vi "MS Auto Operation.vi"() -> ()   [LabVIEW 2016]
uses:
  <vilib>/rvi/interface/nirviReadWriteControl/nirviReadWriteControl.xnode
  <vilib>/rvi/interface/nirviOpenFPGA/nirviOpenFPGA.xnode
  <vilib>/rvi/interface/nirviCloseFPGA/nirviCloseFPGA.xnode
  <vilib>/rvi/interface/nirviMethod/nirviMethod.xnode
  Subsystems/Global Variables.vi
  <vilib>/Analysis/Matrix/Datatypes/RealMatrix.ctl
  <vilib>/Analysis/Matrix/NI_Matrix.lvlib
  NiFpgaLv.dll
  <vilib>/Utility/error.llb/Error Cluster From Error Code.vi
  <vilib>/rvi/errors/niLvFpgaAdjustHostInterfaceError.vi
  IRISS_FPGA_IO_RIO.vi
  FPGA Bitfiles/IRISSTrack_FPGATarget2_IRISSFPGAIORIO_4NTO9ubhv-c.lvbitx
  <vilib>/FPGAPlugInAG/myRIO-1900/niLvFpga_Open_myRIO-1900.vi
  <vilib>/FPGAPlugInAG/myRIO-1900/niLvFpga_Reset_myRIO-1900.vi
  <vilib>/FPGAPlugInAG/myRIO-1900/niLvFpga_Close_myRIO-1900.vi
panel:
  out "Stage PID Cluster":T1={"Stage Z PID"={"Kp"=0.0005, "Kd"=0.001, "Ki"=0.0}, "Stage Y PID"={"Kp"=0.0003, "Kd"=0.01, "Ki"=0.0}, "Stage X PID"={"Kp"=0.0003, "Kd"=0.01, "Ki"=0.0}}
  out "L1 to L4 PID Cluster":T2={"L1 PID Gains"={"Kp"=0.005, "Kd"=0.5, "Ki"=0.0005}, "L2 PID Gains"={"Kp"=0.01, "Kd"=1.0, "Ki"=0.0005}, "L3 PID Gains"={"Kp"=0.05, "Kd"=1.0, "Ki"=0.0005}, "L4 PID Gains"={"Kp"=0.1, "Kd"=1.0, "Ki"=0.0005}}
  in  "IRISS GUI":T3(tab)
  in  "Reroute Hold [sec]":dbl=10.0 caption="Hold [sec]"
  out "X Stage out [mm] 2":dbl caption="Stage X [mm]" format="%#.4f"
  out "Z Stage out [mm] 2":dbl caption="Stage Z [mm]" format="%#.4f"
  out "Y Stage out [mm] 2":dbl caption="Stage Y [mm]" format="%#.4f"
  in  "Refractice Index":dbl=1.35
  out "Asgn Pt Out of Bound":bool caption="Assign Pt OOB"
  out "Finished Late Counts":u16
  out "Emergency alarm":bool
  out "Remote sender engaged":bool
  in  "L2 PID Gains":cluster{"Kp":dbl, "Kd":dbl, "Ki":dbl}={"Kp"=0.01, "Kd"=1.0, "Ki"=0.005}
  in  "L3 PID Gains":cluster{"Kp":dbl, "Kd":dbl, "Ki":dbl}={"Kp"=0.05, "Kd"=1.0, "Ki"=0.0005}
  in  "L4 PID Gains":cluster{"Kp":dbl, "Kd":dbl, "Ki":dbl}={"Kp"=0.1, "Kd"=0.1, "Ki"=0.0005}
  in  "L1 PID Gains":cluster{"Kp":dbl, "Kd":dbl, "Ki":dbl}={"Kp"=0.01, "Kd"=0.5, "Ki"=0.001}
  out "Current System State":T4(ring)
  out "State changing":bool
  out "Current Run No.":u8
  out "Tip out Posit":dbl[](array[numeric]) caption="Position [mm]" format="%#.3f"
  out "Tip cmd Posit":dbl[](array[numeric]) caption="Command [mm]" format="%#.3f"
  out "L4 out Posit":dbl caption="y [deg]" format="%#.2g"
  out "L4 cmd Posit":dbl caption="r [deg]" format="%#.2g"
  out "L3 out Posit":dbl caption="y [mm]" format="%#.2g"
  out "L3 cmd Posit":dbl caption="r [mm]" format="%#.2g"
  out "L2 out Posit":dbl caption="y [deg]" format="%#.2g"
  out "L2 cmd Posit":dbl caption="r [deg]" format="%#.2g"
  out "L1 out Posit":dbl caption="y [deg]" format="%#.2g"
  out "L1 cmd Posit":dbl caption="r [deg]" format="%#.2g"
  out "State Flag Array":bool[](array[boolean])
  out "Timer":i32 format="%<%M:%S>t"
  out "Elaspsed Time":sgl
  in  "File Path":path=path "C:/KevData1.txt"
  in  "Seconds of Data":sgl=5.0
  out "Period [ms]":i64=10
  in  "Remote Control Source":u16(ring) caption="Remote Source" items=["Surgical Console", "Joystick"]
  in  "Reset Joystick":bool caption="Encoder Reset"
  in  "Robot Command":dbl[](array[numeric])=[0.0, 0.0, 0.0, 0.0]
  out "Z Stage out [mm]":dbl caption="Output Z [mm]" format="%#.4f"
  out "Z Stage cmd [mm]":dbl=6.0 caption="Reference Z [mm]" min=0.0 max=12.0 step=0.5
  out "Y Stage out [mm]":dbl caption="Output Y [mm]" format="%#.4f"
  out "Y Stage cmd [mm]":dbl=6.0 caption="Reference Y  [mm]" min=0.0 max=12.0 step=0.5
  out "X Stage out [mm]":dbl caption="Output X [mm]" format="%#.4f"
  out "X Stage cmd [mm]":dbl=6.0 caption="Reference X [mm]" min=0.0 max=12.0 step=0.5
  in  "Stage Z PID Gains":cluster{"Kp":dbl, "Kd":dbl, "Ki":dbl}={"Kp"=0.0005, "Kd"=0.001, "Ki"=0.0}
  in  "Stage Y PID Gains":cluster{"Kp":dbl, "Kd":dbl, "Ki":dbl}={"Kp"=0.0001, "Kd"=0.005, "Ki"=0.0}
  in  "Stage X PID Gains":cluster{"Kp":dbl, "Kd":dbl, "Ki":dbl}={"Kp"=0.0003, "Kd"=0.01, "Ki"=0.0}
  in  "Reroute Transit Vacf":dbl=100.0
  in  "Z Rot Axis":dbl=1.0
  in  "Z Dist Thld":dbl[](array[numeric])=[0.5, 2.0] caption="Z Distance Threshould"
  in  "Vac Extremum":dbl[](array[numeric])=[80.0, 100.0] caption="Vacuum Extremum"
  in  "Min PC Gap":dbl=0.1 caption="Min PC Gap [mm]" min=0.0 max=10.0 step=0.1 format="%#.3g"
  in  "Min AC Gap":dbl=0.1 caption="Min AC Gap [mm]" min=0.0 max=10.0 step=0.1 format="%#.3g"
  in  "Joint Limits":dbl[][](array[numeric])=[[-8.0, 35.0], [-35.0, 35.0], [-5.0, 10.0], [-180.0, 180.0]] format="%#.3g"
  in  "Offset Home 2 RCM":dbl[](array[numeric])=[-7.7, 37.0, 55.0, 0.0] format="%#.3g"
  out "Error(s) Out on Program End":errorcluster
  out "L4 Waveform Graph":dbl[](graph)
  out "L3 Waveform Graph":dbl[](graph)
  out "L2 Waveform Graph":dbl[](graph)
  out "L1 Waveform Graph":dbl[](graph)
  in  "Aiming Pt":dbl[](array[numeric])=[10.0, 0.0, -1.0, 0.0] format="%#.3g"
  in  "Engage Pt":dbl[](array[numeric])=[15.0, 0.0, 3.0, 0.0] format="%#.3g"
  in  "Inc Ctrl":dbl[](array[numeric])=[0.1, 0.05, 0.05] caption="Increment Control"
  in  "L3 Go Home":bool caption="To M/S"
  in  "Program Stop":bool
  # "M/S\n\nAuto"
  # "Robot Status"
  # "Tool Tip Location"
  # "Tracking Planning"
  # "L1"
  # "X\nY\nZ"
  # "X\nY\nZ"
  # "L2"
  # "System Progress"
  # "Assign Point Rerouting"
  # "X\nY\nZ"
  # "L3"
  # "Homing finished"
  # "M/S initialization finished"
  # "Tool Cruising Boundaries"
  # "Trajecoty loading finished"
  # "XY-plane"
  # "Z-axis"
  # "Aiming finished"
  # "L4"
  # "Tool engaged"
  # "Tracking initialization finished"
  # "In Tracking"
  # "Rerouting finished"
  # "In regulation"
  # "Vacuum"
  # "X\nY"
  # "X\nY"
  # "L1"
  # "L2"
  # "L3"
  # "L4"
  # "Data Saving"
  # "IOP Feedback Control"
  # "XYZ Stage Control"
  # "OCT Z-Axis"
  # "Foot Pedal Buttons"
  # "Irrigation and Aspiration"
  # "Button 1"
  # "Button 2"
  # "Button 3"
  # "Rotation & Vacuum Force Scheduling"
  # "Joint Motion & Control"
  # "Calibration"
  # "Space Deform Parameters"
  # "L1"
  # "[deg]"
  # "S"
  # "L2"
  # "[deg]"
  # "R"
  # "[deg]"
  # "L3"
  # "[mm]"
  # "T"
  # "[mm]"
  # "L4"
  # "[deg]"
  # "First Track Point"
  # "AC & PC Gap"
  # "L1"
  # "[deg]"
  # "L2"
  # "[deg]"
  # "L3"
  # "[mm]"
  # "L4"
  # "[deg]"
  # "Error Message"
  # "Tracking Joint Limits"
  # "Incision"
  # "Min."
  # "Max."
  # "L1"
  # "L1"
  # "[deg]"
  # "L2"
  # "L2"
  # "[deg]"
  # "L3"
  # "L3"
  # "[mm]"
  # "L4"
  # "L4"
  # "[deg]"
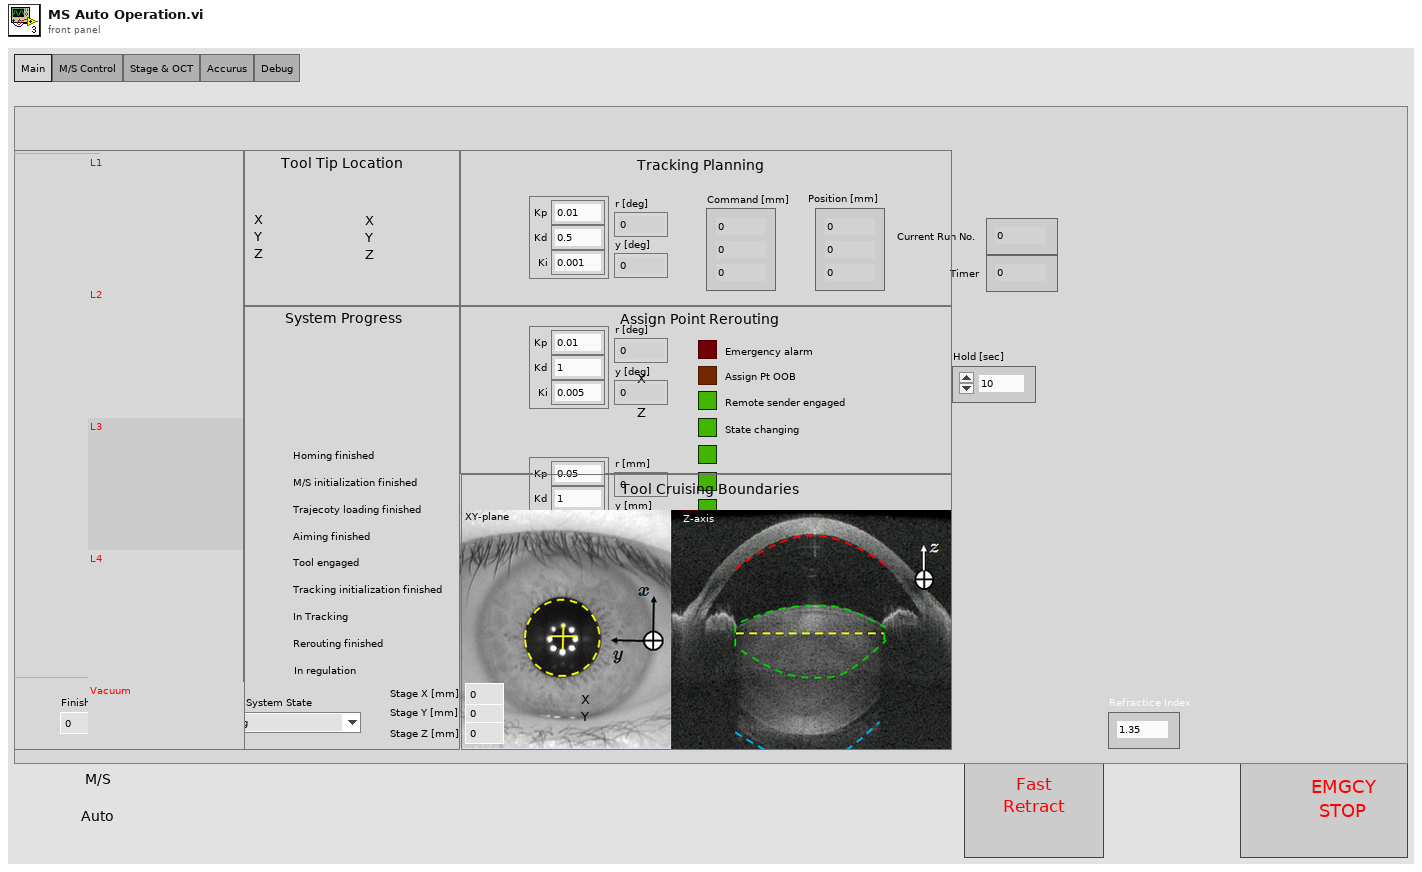
[diagram p1: front panel]
types:
  T1 = cluster{"Stage Z PID":cluster{"Kp":dbl, "Kd":dbl, "Ki":dbl}, "Stage Y PID":cluster{"Kp":dbl, "Kd":dbl, "Ki":dbl}, "Stage X PID":cluster{"Kp":dbl, "Kd":dbl, "Ki":dbl}}
  T2 = cluster{"L1 PID Gains":cluster{"Kp":dbl, "Kd":dbl, "Ki":dbl}, "L2 PID Gains":cluster{"Kp":dbl, "Kd":dbl, "Ki":dbl}, "L3 PID Gains":cluster{"Kp":dbl, "Kd":dbl, "Ki":dbl}, "L4 PID Gains":cluster{"Kp":dbl, "Kd":dbl, "Ki":dbl}}
  T3 = enum32{"Main", "M/S Control", "Stage & OCT", "Accurus", "Debug"}
  T4 = enum16{"Homing", "M/S Initialization", "M/S Operation", "Aiming", "Engaging", "Trajectory Loading", "Tracking Initialization", "Tracking", "Rerouting", "Regulation"}
  T5 = typedef "NI_Matrix.lvlib/RealMatrix.ctl" = dbl[][]
  T6 = cluster{"X Grid":dbl[], "Y Grid":dbl[], "Za_true Surf":dbl[][], "Iris Center":dbl[], "Zp_true Surf":dbl[][], "Pinv":T5, "za_true":dbl, "za_work":dbl, "zp_work":dbl, "zp_true":dbl}
  T7 = cluster{"Traj Px Array":dbl[], "Traj Py Array":dbl[], "Traj Pz Array":dbl[], "Speed Array":dbl[], "Depth Array":dbl[]}
  T8 = cluster{"Prev L1 to L4 Posit":dbl[], "Prev Stage Posit":dbl[], "Prev OCT Z Posit":dbl}
  T9 = cluster{"L1 to L4 PID Cluster":cluster{"L1 PID Gains":cluster{"Kp":dbl, "Kd":dbl, "Ki":dbl}, "L2 PID Gains":cluster{"Kp":dbl, "Kd":dbl, "Ki":dbl}, "L3 PID Gains":cluster{"Kp":dbl, "Kd":dbl, "Ki":dbl}, "L4 PID Gains":cluster{"Kp":dbl, "Kd":dbl, "Ki":dbl}}, "Stage PID Cluster":cluster{"Stage Z PID":cluster{"Kp":dbl, "Kd":dbl, "Ki":dbl}, "Stage Y PID":cluster{"Kp":dbl, "Kd":dbl, "Ki":dbl}, "Stage X PID":cluster{"Kp":dbl, "Kd":dbl, "Ki":dbl}}, "OCT Z PID Gains":cluster{"Kp":dbl, "Kd":dbl, "Ki":dbl}}
  T10 = cluster{"Last L1 to L4 Posit":dbl[], "Last Stage Posit":dbl[], "Last OCT Z Posit":dbl}
  T11 = enum16{"Homing", "M/S Initialization", "M/S Operation"}
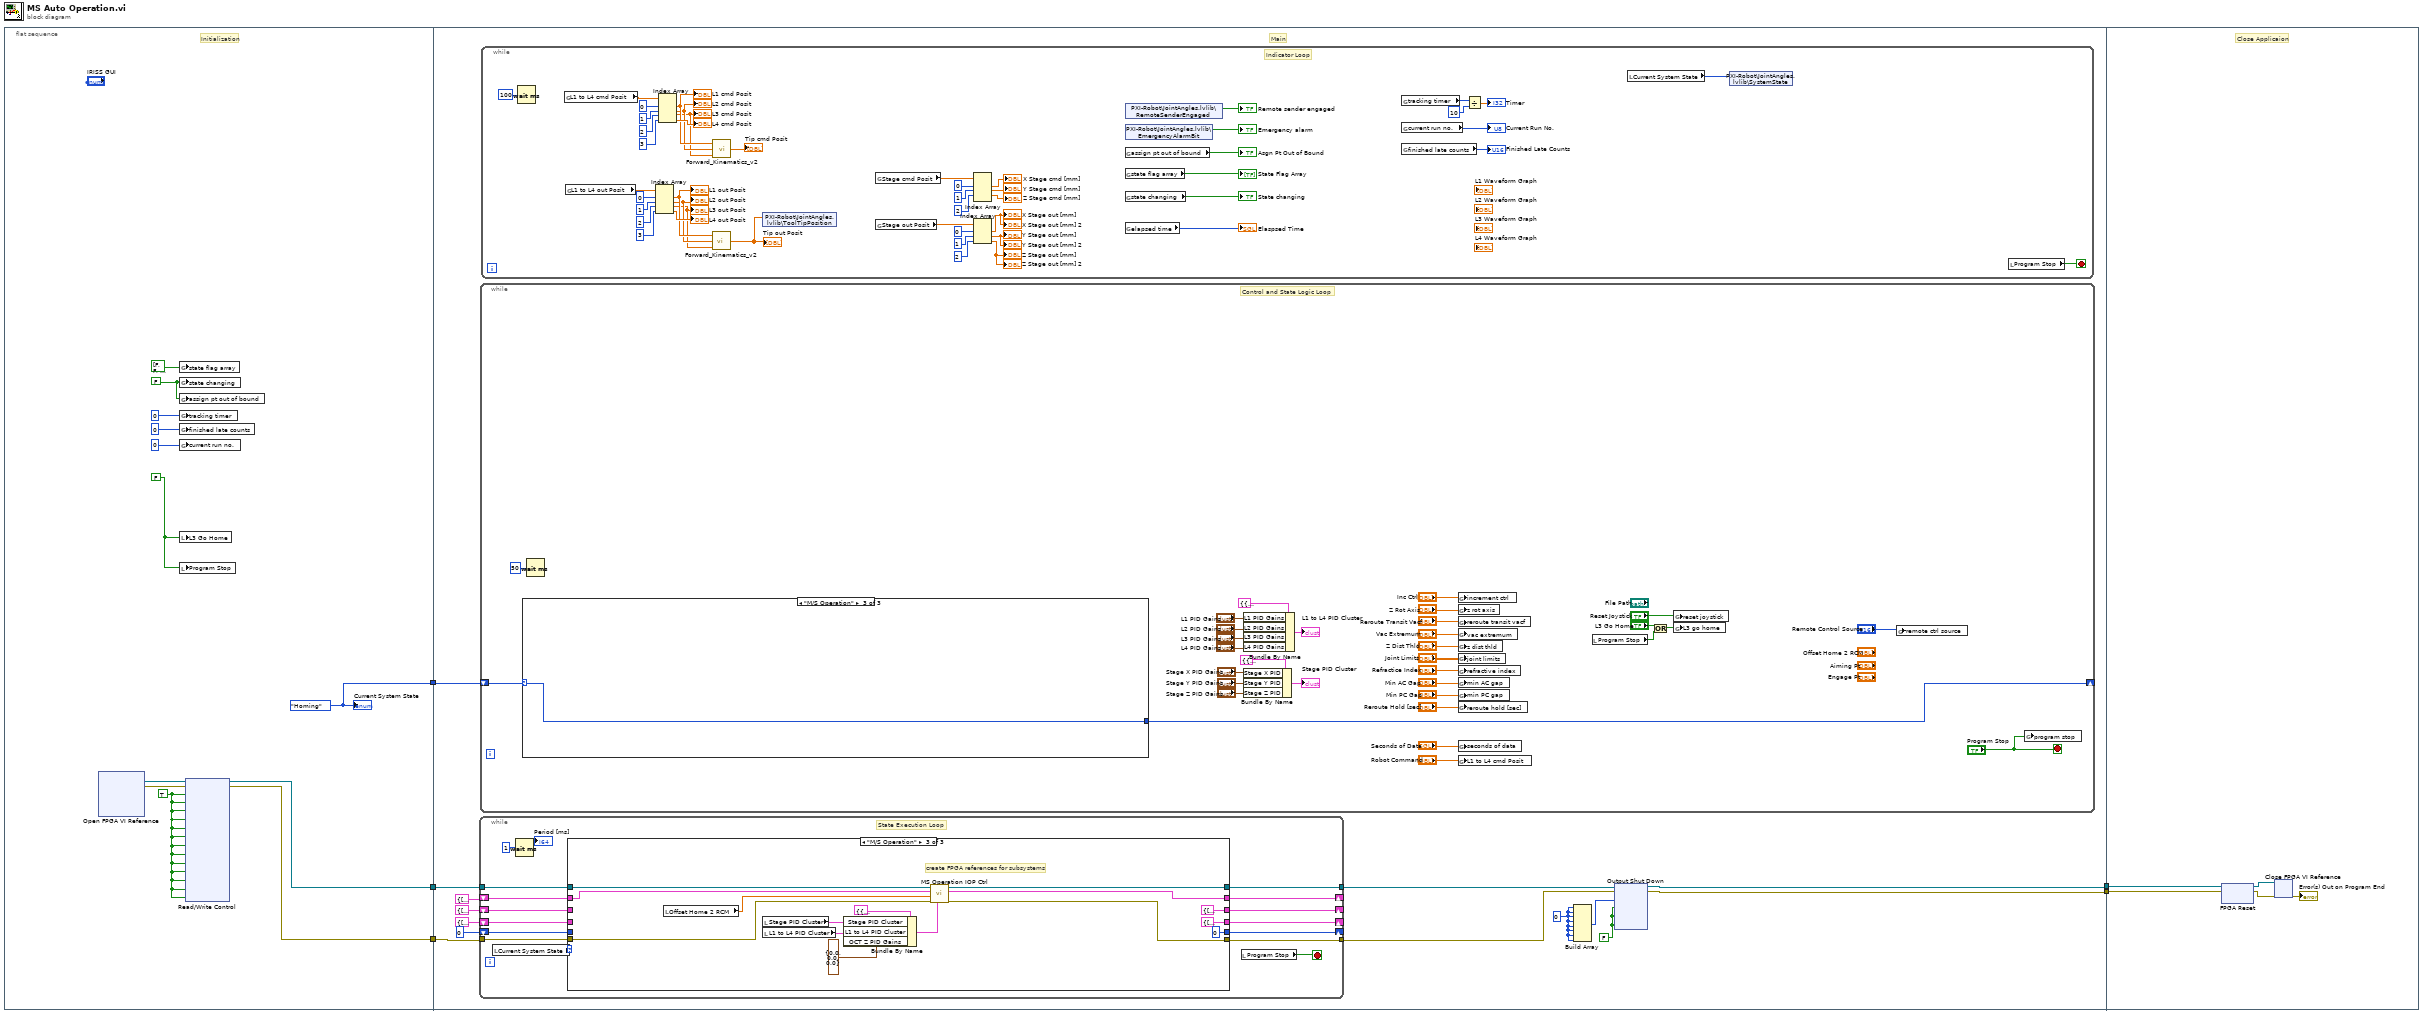
[diagram p0: block diagram]
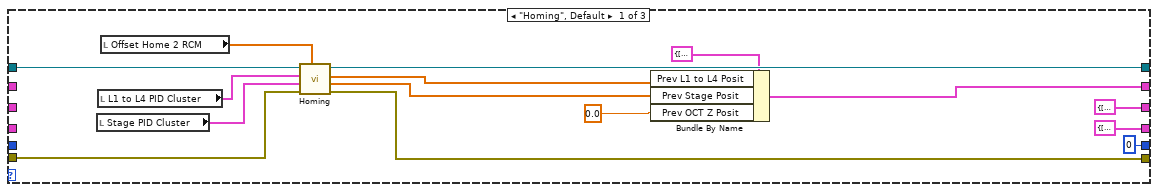
[diagram p2: hidden frame]
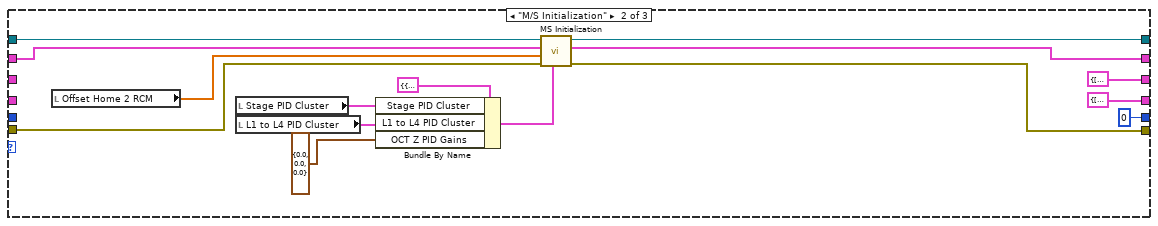
[diagram p3: hidden frame]
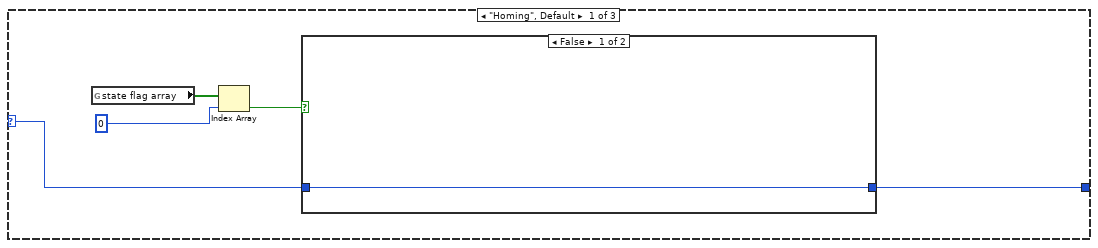
[diagram p4: hidden frame]
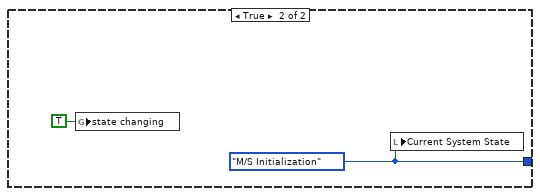
[diagram p5: hidden frame]
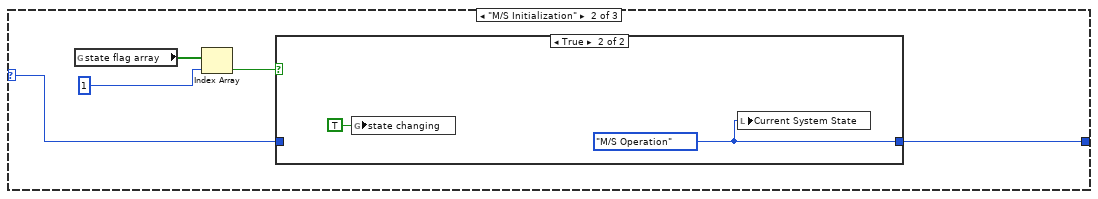
[diagram p6: hidden frame]
diagram:
  n1 = flat-sequence {
    tunnel: [w14] -> w5
    tunnel: [w13] -> w4
    tunnel: [w10] -> w3
    tunnel: w5 -> [w30]
    tunnel: w4 -> [w31]
    tunnel: w3 -> [w22]
    tunnel: [w24] -> w2
    tunnel: [w23] -> w1
    tunnel: w2 -> [w189]
    tunnel: w1 -> [w190]
    frame #0 {
      w10 = T4."Homing" ("Current State")
      w11 = FALSE ("state changing")
      w17 = TRUE ("Reset")
      w6 = FALSE ("program stop")
      # "Initialization"
      n2 = xnode "Open FPGA VI Reference"() -> ("FPGA VI Reference Out"=w16:refnum<k20>, "error out"=w15:errorcluster)  [unwired: 2 in]
      n3 = global write "Global Variables.vi" "state flag array"(bool[] [FALSE, FALSE, FALSE, FALSE, FALSE, FALSE, FALSE, FALSE, FALSE] ("state flag array")) -> ()
      n4 = global write "Global Variables.vi" "state changing"(w11) -> ()
      n5 = global write "Global Variables.vi" "assign pt out of bound"(w11) -> ()
      n6 = global write "Global Variables.vi" "tracking timer"(0 ("finished late counts")) -> ()
      n7 = global write "Global Variables.vi" "finished late counts"(u16 0 ("finished late counts")) -> ()
      n8 = global write "Global Variables.vi" "current run no."(u8 0 ("current run no.")) -> ()
      n9 = local write "L3 Go Home"(w6) -> ()
      n10 = local write "Program Stop"(w6) -> ()
      n11 = xnode "Read/Write Control"("FPGA VI Reference In"=w16, "error in"=w15, "Reset 1"=w17, "Reset 3"=w17, "Reset 9"=w17, "Reset 10"=w17, "Reset 11"=w17, "Reset 12"=w17, "Reset 13"=w17, "Reset 14"=w17, "Reset 15"=w17, "Reset 16"=w17, "Reset 17"=w17, "Reset C1-1"=w17, "Reset C1-4"=w17) -> ("FPGA VI Reference Out"=w13:refnum<k20>, "error out"=w14:errorcluster)
      "Current System State" <- w10
    }
    frame #1 {
      w28 = FALSE
      w20 = i16 0 ("element")
      # "Main"
      n12 = while {
        tunnel: w31 -> [w92]
        tunnel: w30 -> [w91]
        tunnel: [w90] -> w26
        tunnel: [w89] -> w25
        shift-right: [w87] -> _
        shift-left: T8 {"Prev L1 to L4 Posit"=[0.0, 0.0, 0.0, 0.0], "Prev Stage Posit"=[6.0, 6.0, 6.0], "Prev OCT Z Posit"=0.0} ("Prev Posit Cluster") -> [w88]
        shift-right: [w85] -> _
        shift-left: 0 -> [w84]
        shift-right: [w83] -> _
        shift-left: T7 {"Traj Px Array"=[], "Traj Py Array"=[], "Traj Pz Array"=[], "Speed Array"=[], "Depth Array"=[]} ("Trajectory Cluster") -> [w81]
        shift-right: [w82] -> _
        shift-left: T6 {"X Grid"=[], "Y Grid"=[], "Za_true Surf"=[], "Iris Center"=[0.0, 5.0, 0.0], "Zp_true Surf"=[], "Pinv"=[[1.0, 0.0], [0.0, 1.0]], "za_true"=0.0, "za_work"=0.0, "zp_work"=0.0, "zp_true"=0.0} ("Eye Model Cluster") -> [w80]
        stop <- w86 stop-if-true
        # "State Execution Loop"
        n13 = local read "Current System State"() -> (w93:T4)
        n14 = Wait (ms)(milliseconds to wait=u32 1) -> ()  [unwired: 1 out]
        n15 = case shown="\"M/S Operation\"" w93 {
          tunnel: w92 -> [w109 w110 w139]
          tunnel: w91 -> [w108 w124 w138]
          tunnel: [w107 w123 w137] -> w90
          tunnel: [w106 w122 w136] -> w89
          tunnel: w88 -> [_ w121 w135]
          tunnel: [w105 w120 w134] -> w87
          tunnel: [0 ("Last Index") 0 ("Last Index") 0 ("Last Index")] -> w85
          tunnel: w84 -> [_ _ _]
          tunnel: [T7 {"Traj Px Array"=[], "Traj Py Array"=[], "Traj Pz Array"=[], "Speed Array"=[], "Depth Array"=[]} ("Trajectory Cluster") T7 {"Traj Px Array"=[], "Traj Py Array"=[], "Traj Pz Array"=[], "Speed Array"=[], "Depth Array"=[]} ("Trajectory Cluster") T7 {"Traj Px Array"=[], "Traj Py Array"=[], "Traj Pz Array"=[], "Speed Array"=[], "Depth Array"=[]} ("Trajectory Cluster")] -> w83
          tunnel: [T6 {"X Grid"=[], "Y Grid"=[], "Za_true Surf"=[], "Iris Center"=[0.0, 5.0, 0.0], "Zp_true Surf"=[], "Pinv"=[[1.0, 0.0], [0.0, 1.0]], "za_true"=0.0, "za_work"=0.0, "zp_work"=0.0, "zp_true"=0.0} ("Eye Model Cluster") T6 {"X Grid"=[], "Y Grid"=[], "Za_true Surf"=[], "Iris Center"=[0.0, 5.0, 0.0], "Zp_true Surf"=[], "Pinv"=[[1.0, 0.0], [0.0, 1.0]], "za_true"=0.0, "za_work"=0.0, "zp_work"=0.0, "zp_true"=0.0} ("Eye Model Cluster") T6 {"X Grid"=[], "Y Grid"=[], "Za_true Surf"=[], "Iris Center"=[0.0, 5.0, 0.0], "Zp_true Surf"=[], "Pinv"=[[1.0, 0.0], [0.0, 1.0]], "za_true"=0.0, "za_work"=0.0, "zp_work"=0.0, "zp_true"=0.0} ("Eye Model Cluster")] -> w82
          tunnel: w81 -> [_ _ _]
          tunnel: w80 -> [_ _ _]
          frame "Homing", Default {
            n16 = local read "Stage PID Cluster"() -> (w101:T1)
            n17 = local read "L1 to L4 PID Cluster"() -> (w102:T2)
            n18 = local read "Offset Home 2 RCM"() -> (w104:dbl[])
            n19 = call "Homing.vi"("Offset Home 2 RCM"=w104, "error in"=w108, "Stage PID Cluster"=w101, "L1 to L4 PID Cluster"=w102, "FPGA VI Reference In"=w109) -> ("error out"=w106:errorcluster, "Last Stage Posit"=w98:dbl[], "Last L1 to L4 Posit"=w99:dbl[], "FPGA VI Reference Out"=w107:refnum<k20>)  [unwired: 3 in]
            n20 = Bundle By Name(cluster=T8 {"Prev L1 to L4 Posit"=[-0.5409, 0.04404050915429177, -1.917656453185038, 0.02068014705882353], "Prev Stage Posit"=[6.001471972029684, 5.996134588585126, 6.000298217087839], "Prev OCT Z Posit"=-0.0} ("Prev Posit Cluster"), "Prev L1 to L4 Posit"=w99, "Prev Stage Posit"=w98, "Prev OCT Z Posit"=0.0) -> (w105:T8)
          }
          frame "M/S Initialization" {
            n21 = local read "Offset Home 2 RCM"() -> (w115:dbl[])
            n22 = local read "Stage PID Cluster"() -> (w119:T1)
            n23 = local read "L1 to L4 PID Cluster"() -> (w118:T2)
            n24 = Bundle By Name(cluster=T9 {"L1 to L4 PID Cluster"={"L1 PID Gains"={"Kp"=0.005, "Kd"=0.5, "Ki"=0.0005}, "L2 PID Gains"={"Kp"=0.01, "Kd"=1.0, "Ki"=0.005}, "L3 PID Gains"={"Kp"=0.05, "Kd"=1.0, "Ki"=0.0005}, "L4 PID Gains"={"Kp"=0.1, "Kd"=0.1, "Ki"=0.0005}}, "Stage PID Cluster"={"Stage Z PID"={"Kp"=0.0005, "Kd"=0.001, "Ki"=0.0}, "Stage Y PID"={"Kp"=0.0003, "Kd"=0.01, "Ki"=0.0}, "Stage X PID"={"Kp"=0.0003, "Kd"=0.01, "Ki"=0.0}}, "OCT Z PID Gains"={"Kp"=0.0003, "Kd"=0.0001, "Ki"=0.01}} ("PID Cluster"), "Stage PID Cluster"=w119, "L1 to L4 PID Cluster"=w118, "OCT Z PID Gains"=cluster{"Kp":dbl, "Kd":dbl, "Ki":dbl} {"Kp"=0.0, "Kd"=0.0, "Ki"=0.0}) -> (w116:T9)
            n25 = call "MS Initialization.vi"("PID Cluster"=w116, "error in"=w124, "Offset Home 2 RCM"=w115, "Prev Posit Cluster"=w121, "FPGA VI Reference In"=w110) -> ("error out"=w122:errorcluster, "Last Posit Cluster"=w120:T10, "FPGA VI Reference Out"=w123:refnum<k20>)  [unwired: 4 in]
          }
          frame "M/S Operation" {
            # "create FPGA references for subsystems"
            n26 = local read "Offset Home 2 RCM"() -> (w129:dbl[])
            n27 = local read "Stage PID Cluster"() -> (w133:T1)
            n28 = local read "L1 to L4 PID Cluster"() -> (w132:T2)
            n29 = Bundle By Name(cluster=T9 {"L1 to L4 PID Cluster"={"L1 PID Gains"={"Kp"=0.005, "Kd"=0.5, "Ki"=0.0005}, "L2 PID Gains"={"Kp"=0.01, "Kd"=1.0, "Ki"=0.005}, "L3 PID Gains"={"Kp"=0.05, "Kd"=1.0, "Ki"=0.0005}, "L4 PID Gains"={"Kp"=0.1, "Kd"=0.1, "Ki"=0.0005}}, "Stage PID Cluster"={"Stage Z PID"={"Kp"=0.0005, "Kd"=0.001, "Ki"=0.0}, "Stage Y PID"={"Kp"=0.0003, "Kd"=0.01, "Ki"=0.0}, "Stage X PID"={"Kp"=0.0003, "Kd"=0.01, "Ki"=0.0}}, "OCT Z PID Gains"={"Kp"=0.0003, "Kd"=0.0001, "Ki"=0.01}} ("PID Cluster"), "Stage PID Cluster"=w133, "L1 to L4 PID Cluster"=w132, "OCT Z PID Gains"=cluster{"Kp":dbl, "Kd":dbl, "Ki":dbl} {"Kp"=0.0, "Kd"=0.0, "Ki"=0.0}) -> (w130:T9)
            n30 = call "MS Operation IOP Ctrl.vi"("PID Cluster"=w130, "error in"=w138, "Offset Home 2 RCM"=w129, "Prev Posit Cluster"=w135, "FPGA VI Reference In"=w139) -> ("error out"=w136:errorcluster, "Last Posit Cluster"=w134:T10, "FPGA VI Reference Out"=w137:refnum<k20>)  [unwired: 4 in]
          }
        }
        n31 = local read "Program Stop"() -> (w86:bool)
      }
      n32 = while {
        shift-right: [w148] -> _
        shift-left: w22 -> [w149]
        stop <- "Program Stop" stop-if-true
        # "Control and State Logic Loop"
        n33 = case shown="\"M/S Operation\"" w149 {
          selector: w149 -> [w174 w180 w188]
          tunnel: [w173 w181 w188] -> w148
          frame "Homing", Default {
            n34 = global read "Global Variables.vi" "state flag array"() -> (w175:bool[])
            n35 = Index Array(array=w175, index=0) -> (element=w172:bool)
            n36 = case shown="False" w172 {
              tunnel: [w177 w178] -> w173
              tunnel: w174 -> [w177 _]
              frame False {
                # "homing in process"
              }
              frame True {
                w178 = T4."M/S Initialization" ("Current State")
                # "finish homing"
                n37 = global write "Global Variables.vi" "state changing"(TRUE ("state changing")) -> ()
                n38 = local write "Current System State"(w178) -> ()
              }
            }
          }
          frame "M/S Initialization" {
            n39 = global read "Global Variables.vi" "state flag array"() -> (w183:bool[])
            n40 = Index Array(array=w183, index=1) -> (element=w182:bool)
            n41 = case shown="True" w182 {
              tunnel: [w185 w186] -> w181
              tunnel: w180 -> [w185 _]
              frame False {
              }
              frame True {
                w186 = T11."M/S Operation" ("Current State")
                n42 = global write "Global Variables.vi" "state changing"(TRUE ("state changing")) -> ()
                n43 = local write "Current System State"(w186) -> ()
              }
            }
          }
          frame "M/S Operation" {
          }
        }
        n44 = Wait (ms)(milliseconds to wait=u32 50) -> ()  [unwired: 1 out]
        n45 = Bundle By Name(cluster=T2 {"L1 PID Gains"={"Kp"=0.005, "Kd"=0.5, "Ki"=0.0005}, "L2 PID Gains"={"Kp"=0.01, "Kd"=1.0, "Ki"=0.0005}, "L3 PID Gains"={"Kp"=0.05, "Kd"=1.0, "Ki"=0.0005}, "L4 PID Gains"={"Kp"=0.1, "Kd"=1.0, "Ki"=0.0005}} ("L1 to L4 PID Cluster 2"), "L1 PID Gains"="L1 PID Gains", "L2 PID Gains"="L2 PID Gains", "L3 PID Gains"="L3 PID Gains", "L4 PID Gains"="L4 PID Gains") -> (→"L1 to L4 PID Cluster":T2)
        n46 = Bundle By Name(cluster=T1 {"Stage Z PID"={"Kp"=0.0005, "Kd"=0.001, "Ki"=0.0}, "Stage Y PID"={"Kp"=0.0003, "Kd"=0.01, "Ki"=0.0}, "Stage X PID"={"Kp"=0.0003, "Kd"=0.01, "Ki"=0.0}} ("Stage PID Cluster 2"), "Stage X PID"="Stage X PID Gains", "Stage Y PID"="Stage Y PID Gains", "Stage Z PID"="Stage Z PID Gains") -> (→"Stage PID Cluster":T1)
        n47 = global write "Global Variables.vi" "increment ctrl"("Inc Ctrl") -> ()
        n48 = global write "Global Variables.vi" "z rot axis"("Z Rot Axis") -> ()
        n49 = global write "Global Variables.vi" "reroute transit vacf"("Reroute Transit Vacf") -> ()
        n50 = global write "Global Variables.vi" "vac extremum"("Vac Extremum") -> ()
        n51 = global write "Global Variables.vi" "z dist thld"("Z Dist Thld") -> ()
        n52 = global write "Global Variables.vi" "joint limits"("Joint Limits") -> ()
        n53 = global write "Global Variables.vi" "refractive index"("Refractice Index") -> ()
        n54 = global write "Global Variables.vi" "min AC gap"("Min AC Gap") -> ()
        n55 = global write "Global Variables.vi" "min PC gap"("Min PC Gap") -> ()
        n56 = global write "Global Variables.vi" "reroute hold [sec]"("Reroute Hold [sec]") -> ()
        n57 = global write "Global Variables.vi" "seconds of data"("Seconds of Data") -> ()
        n58 = global write "Global Variables.vi" "L1 to L4 cmd Posit"("Robot Command") -> ()
        n59 = local read "Program Stop"() -> (w152:bool)
        n60 = Or(x="L3 Go Home", y=w152) -> (x .or. y?=w153:bool)
        n61 = global write "Global Variables.vi" "reset joystick"("Reset Joystick") -> ()
        n62 = global write "Global Variables.vi" "L3 go home"(w153) -> ()
        n63 = global write "Global Variables.vi" "remote ctrl source"("Remote Control Source") -> ()
        n64 = global write "Global Variables.vi" "program stop"("Program Stop") -> ()
      }
      n65 = while {
        stop <- w59 stop-if-true
        # "Indicator Loop"
        n66 = Wait (ms)(milliseconds to wait=u32 100) -> ()  [unwired: 1 out]
        n67 = global read "Global Variables.vi" "L1 to L4 cmd Posit"() -> (w48:dbl[])
        n68 = global read "Global Variables.vi" "L1 to L4 out Posit"() -> (w51:dbl[])
        n69 = Index Array(array=w51, index #1=0 ("index"), index #2=1 ("index"), index #3=2 ("index"), index #4=3 ("index")) -> (element #1=w54:dbl, element #2=w53:dbl, element #3=w52:dbl, element #4=→"L4 out Posit":dbl)
        "L3 out Posit" <- w52
        "L2 out Posit" <- w53
        "L1 out Posit" <- w54
        n70 = Index Array(array=w48, index #1=0 ("index"), index #2=1 ("index"), index #3=2 ("index"), index #4=3 ("index")) -> (element #1=w58:dbl, element #2=w57:dbl, element #3=w56:dbl, element #4=→"L4 cmd Posit":dbl)
        "L1 cmd Posit" <- w58
        "L3 cmd Posit" <- w56
        "L2 cmd Posit" <- w57
        n71 = call "Forward_Kinematics_v2.vi"("theta 3"=w52, "theta 2"=w53, "theta 1"=w54) -> ("position"=w44:dbl[])
        "Tip out Posit" <- w44
        n72 = call "Forward_Kinematics_v2.vi"("theta 3"=w56, "theta 2"=w57, "theta 1"=w58) -> ("position"=→"Tip cmd Posit":dbl[])
        n73 = shared-variable "PXI-Robot\\JointAngles.lvlib\\ToolTipPosition"(w44) -> ()  [unwired: 1 in, 1 out]
        n74 = global read "Global Variables.vi" "Stage cmd Posit"() -> (w49:dbl[])
        n75 = global read "Global Variables.vi" "Stage out Posit"() -> (w50:dbl[])
        n76 = Index Array(array=w50, index #1=0 ("index"), index #2=1 ("index"), index #3=2 ("index")) -> (element #1=→"X Stage out [mm]" →"X Stage out [mm] 2":dbl, element #2=→"Y Stage out [mm]" →"Y Stage out [mm] 2":dbl, element #3=→"Z Stage out [mm]" →"Z Stage out [mm] 2":dbl)
        n77 = Index Array(array=w49, index #1=0 ("index"), index #2=1 ("index"), index #3=2 ("index")) -> (element #1=→"X Stage cmd [mm]":dbl, element #2=→"Y Stage cmd [mm]":dbl, element #3=→"Z Stage cmd [mm]":dbl)  [unwired: 1 in, 1 out]
        n78 = shared-variable "PXI-Robot\\JointAngles.lvlib\\RemoteSenderEngaged"() -> (→"Remote sender engaged":bool)  [unwired: 1 in, 1 out]
        n79 = shared-variable "PXI-Robot\\JointAngles.lvlib\\EmergencyAlarmBit"() -> (→"Emergency alarm":bool)  [unwired: 1 in, 1 out]
        n80 = global read "Global Variables.vi" "assign pt out of bound"() -> (→"Asgn Pt Out of Bound":bool)
        n81 = global read "Global Variables.vi" "state flag array"() -> (→"State Flag Array":bool[])
        n82 = global read "Global Variables.vi" "state changing"() -> (→"State changing":bool)
        n83 = global read "Global Variables.vi" "elapsed time"() -> (→"Elaspsed Time":u16)
        n84 = global read "Global Variables.vi" "tracking timer"() -> (w39:i32)
        n85 = global read "Global Variables.vi" "current run no."() -> (→"Current Run No.":u8)
        n86 = global read "Global Variables.vi" "finished late counts"() -> (→"Finished Late Counts":u16)
        n87 = Divide(x=w39, y=10) -> (x/y=→"Timer":dbl)
        n88 = local read "Current System State"() -> (w33:T4)
        n89 = shared-variable "PXI-Robot\\JointAngles.lvlib\\SystemState"(w33) -> ()  [unwired: 1 in, 1 out]
        n90 = local read "Program Stop"() -> (w59:bool)
      }
      n91 = Build Array(w20, w20, w20, w20, w20, w20, w20, w20) -> (w27:i16[])
      n92 = xnode "Output Shut Down"("FPGA VI Reference In"=w26, "error in"=w25, "AO"=w27, "INHB X"=w28, "INHB Y"=w28, "INHB Z"=w28) -> ("FPGA VI Reference Out"=w23:refnum<k20>, "error out"=w24:errorcluster)
    }
    frame #2 {
      # "Close Applicaion"
      n93 = xnode "FPGA Reset"("FPGA VI Reference In"=w190, "error in"=w189) -> ("FPGA VI Reference Out"=w193:refnum<k20>, "error out"=w192:errorcluster)
      n94 = xnode "Close FPGA VI Reference"("FPGA VI Reference In"=w193, "error in"=w192) -> ("error out"=→"Error(s) Out on Program End":errorcluster)
    }
  }
